vi "WPI_DashboardSave DB Images.vi"(7 "Save Info":T1={"Save Path"=path "", "Interval (s)"=1.0, "Keep"=180}, 8 "Camera Name":string="Camera ", 9 "Image":T2) -> ()   [LabVIEW 2025]
doc: "This VI saves the most recent images at a specified interval. It saves them to the provided path or to the public documents/FRC/DV Images directory. The name is composed of the camera name and the image sequence number."
uses:
  <vilib>/vision/Image Controls.llb/IMAQ Image.ctl
  <vilib>/Utility/sysdir.llb/System Directory Type.ctl
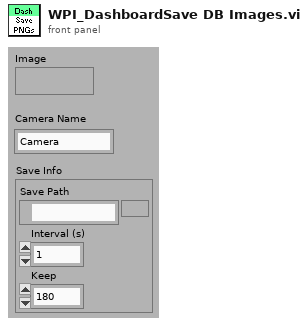
[diagram p1: front panel]
types:
  T1 = cluster{"Save Path":path, "Interval (s)":dbl, "Keep":i32}
  T2 = typedef "IMAQ Image.ctl" = refnum<image>
  T3 = typedef "System Directory Type.ctl" = i32
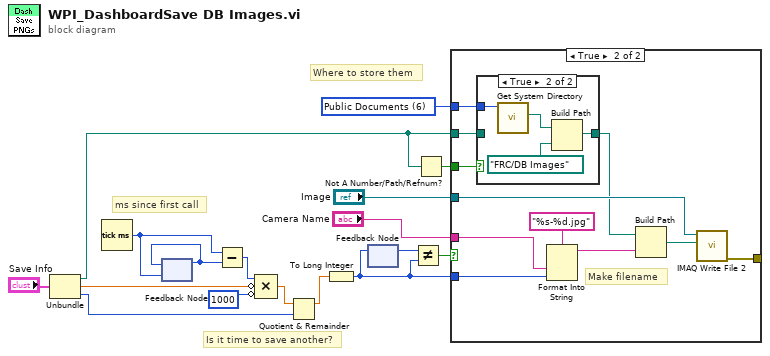
[diagram p0: block diagram]
diagram:
  w7 = T3 6 items=["User Home"=0, "User Desktop"=1, "User Documents"=2, "User Application Data"=3, "User Preferences"=4, "User Temporary"=5, "Public Documents"=6, "Public Application Data"=7, "Public Preferences"=8, "Public Cache"=13, "System Core Libraries"=9, "System Installed Libraries"=10, "Application Files"=11, "Boot Volume Root"=12] ("system directory type")
  # "Where to store them"
  # "Is it time to save another?"
  # "ms since first call"
  n1 = Unbundle("Save Info") -> ("Save Path"=w3:path, "Interval (s)"=w2:dbl, "Keep"=w4:i32)
  n2 = Tick Count (ms)() -> (millisecond timer value=w13:u32)
  n3 = feedback #1(w13) -> (w12:u32)
  n4 = feedback-in #1(w12) -> ()
  n5 = Subtract(x=w13, y=w12) -> (x-y=w15:u32)
  n6 = Compound Arithmetic op=MULTIPLY(w15, invert w2, invert 1000) -> (w10:dbl)
  n7 = Quotient & Remainder(x=w10, y=w4) -> (x-y*floor(x/y)=w9:dbl)  [unwired: 1 out]
  n8 = To Long Integer(number=w9) -> (32bit integer=w11:i32)
  n9 = feedback-in #2(w11) -> ()
  n10 = feedback #2() -> (w16:i32)  [unwired: 1 out]
  n11 = Not Equal?(x=w16, y=w11) -> (x != y?=w17:bool)
  n12 = Not A Number/Path/Refnum?(number/path/refnum=w3) -> (NaN/Path/Refnum?=w8:bool)
  n13 = case shown="True" w17 {
    tunnel: "Image" -> [_ w28]
    tunnel: [_ w26] -> _
    tunnel: w11 -> [_ w19]
    tunnel: w8 -> [_ w24]
    tunnel: w3 -> [_ w23]
    tunnel: w7 -> [_ w21]
    tunnel: "Camera Name" -> [_ w18]
    frame False {
    }
    frame True {
      # "Make filename"
      n14 = case shown="True" w24 {
        tunnel: w23 -> [w29 _]
        tunnel: [w29 w33] -> w22
        tunnel: w21 -> [_ w32]
        frame False {
        }
        frame True {
          n15 = call <vilib>:"Get System Directory.vi"("system directory type"=w32) -> ("system directory"=w31:path)  [unwired: 10 in]
          n16 = Build Path(base path=w31, name or relative path=path "FRC/DB Images") -> (appended path=w33:path)
        }
      }
      n17 = Format Into String(format string="%s-%d.jpg", w18, w19) -> (resulting string=w25:string)  [unwired: 2 in, 1 out]
      n18 = Build Path(base path=w22, name or relative path=w25) -> (appended path=w27:path)
      n19 = call-poly "IMAQ Write File 2"("File Path"=w27, "Image"=w28) -> ("error out"=w26:errorcluster)  [unwired: 3 in, 6 out]
    }
  }
